vi "Table_Check_Creat.vi"(9 "_datetime":string, 11 "pathcheck选项":T1) -> (0 "tablename":string, 2 "table存在？":bool, 3 "database路径":path)   [LabVIEW 2017]
uses:
  Sqlite/CBB/CreatTable.vi
  Sqlite/SQLite.lvlib
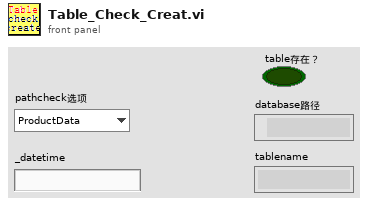
[diagram p1: front panel]
types:
  T1 = typedef "pathcheck选项.ctl" = enum16{"ProductData", "CTData", "ERData", "IOTDATA"}
  T2 = typedef "data格式选项.ctl" = enum16{"生成格式", "加载格式"}
  T3 = typedef "表头集合.ctl" = cluster{"product信息":T4, "CT信息":T5, "ER信息":T6, "IOT信息":T7}
  T4 = typedef "product信息.ctl" = cluster{"product表头整合":string[], "量测部分表头":string[], "前侧贴合表头":string[], "后侧贴合表头":string[]}
  T5 = typedef "CT信息.ctl" = cluster{"CT表头整合":string[], "量测CT":string[], "动子1_2CT":string[], "动子3_4CT":string[]}
  T6 = typedef "ER信息.ctl" = cluster{"ER表头整合":string[]}
  T7 = typedef "IOT信息.ctl" = cluster{"IOT表头整合":string[]}
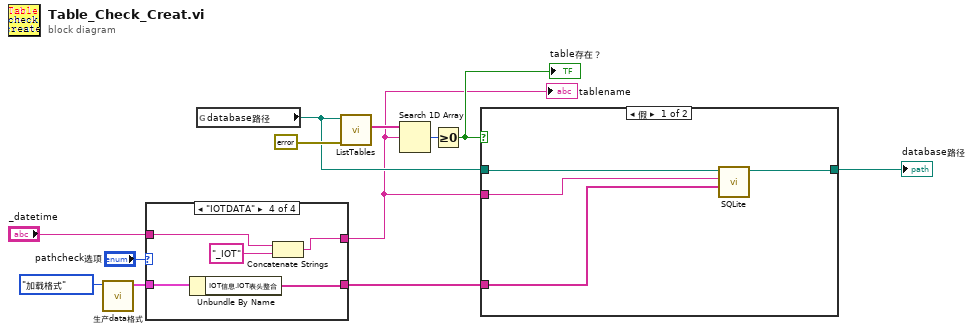
[diagram p0: block diagram]
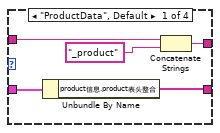
[diagram p2: hidden frame]
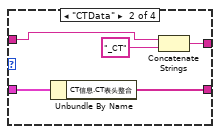
[diagram p3: hidden frame]
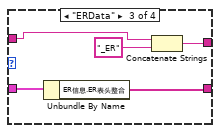
[diagram p4: hidden frame]
diagram:
  n1 = call "生产data格式.vi"("data格式选项"=data格式选项."加载格式") -> ("表头格式"=w3:T3)  [unwired: 10 in]
  n2 = case shown="\"IOTDATA\"" "pathcheck选项" {
    tunnel: "_datetime" -> [w17 w21 w26 w31]
    tunnel: [w15 w20 w24 w30] -> w4
    tunnel: w3 -> [w14 w19 w25 w29]
    tunnel: [w13 w18 w23 w28] -> w2
    frame "ProductData", Default {
      n3 = Unbundle By Name(w14) -> ("product信息.product表头整合"=w13:string[])
      n4 = Concatenate Strings(w17, "_product" ("字符串")) -> (w15:string)
    }
    frame "CTData" {
      n5 = Unbundle By Name(w19) -> ("CT信息.CT表头整合"=w18:string[])
      n6 = Concatenate Strings(w21, "_CT" ("字符串")) -> (w20:string)
    }
    frame "ERData" {
      n7 = Unbundle By Name(w25) -> ("ER信息.ER表头整合"=w23:string[])
      n8 = Concatenate Strings(w26, "_ER" ("字符串")) -> (w24:string)
    }
    frame "IOTDATA" {
      n9 = Unbundle By Name(w29) -> ("IOT信息.IOT表头整合"=w28:string[])
      n10 = Concatenate Strings(w31, "_IOT" ("字符串")) -> (w30:string)
    }
  }
  "tablename" <- w4
  n11 = global read "数据库全局.vi" "database路径"() -> (w8:path)
  n12 = call "ListTables.vi"("error in (no error)"=errorcluster {"status"=FALSE, "code"=0, "source"=""}, "DbPath"=w8) -> ("Tables"=w11:string[])  [unwired: 6 in, 3 out]
  n13 = Search 1D Array(1D array=w11, element=w4) -> (index of element=w10:i32)  [unwired: 1 in]
  n14 = Greater Or Equal To 0?(x=w10) -> (x >= 0?=w9:bool)
  "table存在？" <- w9
  n15 = case shown="假" w9 {
    tunnel: w8 -> [w36 w37]
    tunnel: w4 -> [w35 _]
    tunnel: [w34 w37] -> w7
    tunnel: w2 -> [w33 _]
    frame False {
      n16 = call-poly "SQLite.vi"("Columns"=w33, "Table Name"=w35, "DbPath"=w36) -> ("DbPath out"=w34:path)  [unwired: 6 in, 2 out]
    }
    frame True {
    }
  }
  "database路径" <- w7
